vi "9-1.vi"() -> ()   [LabVIEW 2019, in "9.lvlib"]
uses:
  9.lvlib
panel:
  out "number":i32[][](array[numeric])
  out "sum":i32
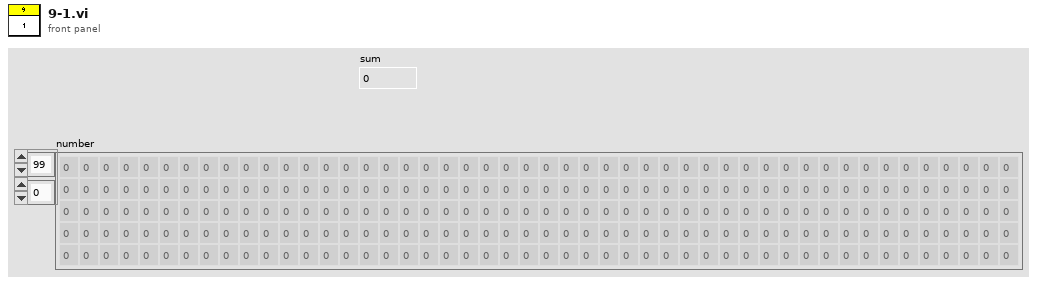
[diagram p1: front panel]
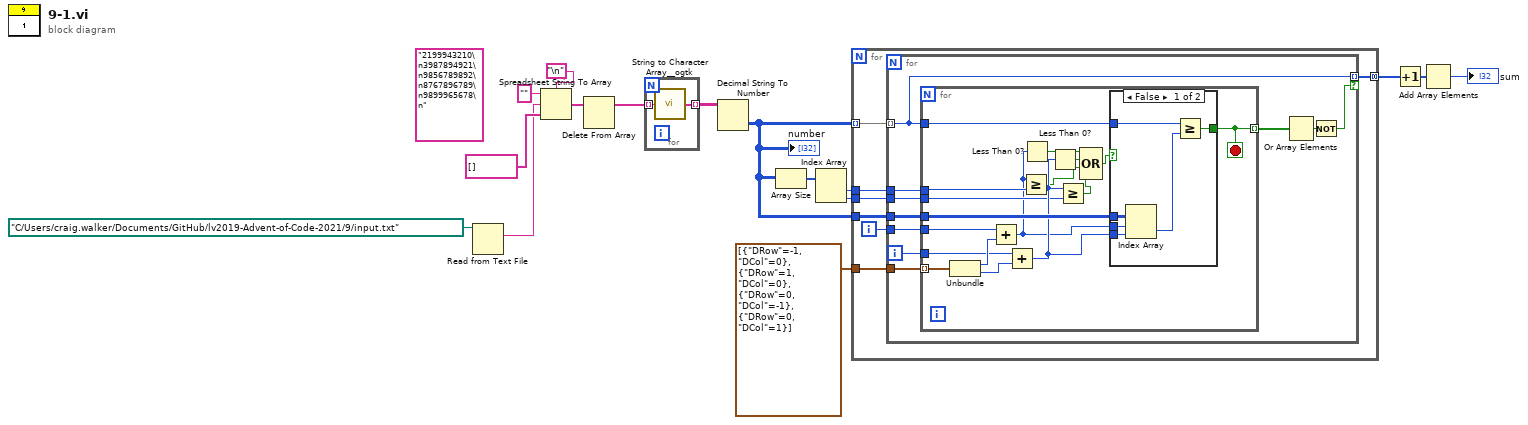
[diagram p0: block diagram]
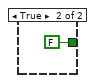
[diagram p2: hidden frame]
diagram:
  (unwired) "2199943210\n3987894921\n9856789892\n8767896789\n9899965678\n"
  n1 = Read from Text File(file (use dialog)=path "C:/Users/craig.walker/Documents/GitHub/lv2019-Advent-of-Code-2021/9/input.txt") -> (text=w1:string)  [unwired: 3 in, 3 out]
  n2 = Spreadsheet String To Array(delimiter (Tab)="\n", format string="", spreadsheet string=w1, array type (2D Dbl)=string[] []) -> (array=w15:string[])
  n3 = Delete From Array(array=w15) -> (array with subset deleted=w2:string[])  [unwired: 2 in, 1 out]
  n4 = for {
    tunnel: w2 -> [w18] mode=indexing
    tunnel: [w17] -> w13 mode=indexing
    n5 = call <userlib>:"String to Character Array__ogtk.vi"("Input String"=w18) -> ("Character Array"=w17:string[])
  }
  n6 = Decimal String To Number(string=w13) -> (number=w3:i32[][])  [unwired: 2 in, 1 out]
  "number" <- w3
  n7 = Array Size(array=w3) -> (size(s)=w7:i32[])
  n8 = Index Array(array=w7) -> (element #1=w9:i32, element #2=w8:i32)  [unwired: 2 in]
  n9 = for {
    tunnel: w3 -> [w24] mode=indexing
    tunnel: w3 -> [w25]
    tunnel: w9 -> [w22]
    tunnel: w8 -> [w21]
    tunnel: cluster{"DRow":i32, "DCol":i32}[] [{"DRow"=-1, "DCol"=0}, {"DRow"=1, "DCol"=0}, {"DRow"=0, "DCol"=-1}, {"DRow"=0, "DCol"=1}] -> [w20]
    tunnel: [w19] -> w12 mode=concatenating
    i -> [w23]
    n10 = for {
      tunnel: w25 -> [w35]
      tunnel: w24 -> [w32] mode=indexing
      tunnel: w23 -> [w28]
      tunnel: w22 -> [w29]
      tunnel: w21 -> [w30]
      tunnel: w20 -> [w34]
      tunnel: [w32] -> w19 mode=indexing if=w26
      i -> [w27]
      n11 = for {
        tunnel: w35 -> [w44]
        tunnel: w28 -> [w50]
        tunnel: w27 -> [w48]
        tunnel: w34 -> [w52] mode=indexing
        tunnel: w32 -> [w42]
        tunnel: [w43] -> w33 mode=indexing
        tunnel: w30 -> [w40]
        tunnel: w29 -> [w39]
        stop <- w43 stop-if-true
        n12 = Unbundle(w52) -> ("DRow"=w51:i32, "DCol"=w49:i32)
        n13 = Add(x=w50, y=w51) -> (x+y=w38:i32)
        n14 = Add(x=w48, y=w49) -> (x+y=w41:i32)
        n15 = Greater Or Equal?(x=w38, y=w39) -> (x >= y?=w37:bool)
        n16 = Less Than 0?(x=w38) -> (x < 0?=w46:bool)
        n17 = Less Than 0?(x=w41) -> (x < 0?=w47:bool)
        n18 = Greater Or Equal?(x=w41, y=w40) -> (x >= y?=w36:bool)
        n19 = Compound Arithmetic op=OR(w46, w47, w37, w36) -> (w45:bool)
        n20 = case shown="False" w45 {
          tunnel: w42 -> [w58 _]
          tunnel: w44 -> [w57 _]
          tunnel: w38 -> [w56 _]
          tunnel: w41 -> [w55 _]
          tunnel: [w53 FALSE] -> w43
          frame False {
            n21 = Index Array(array=w57, index (row)=w56, index (col)=w55) -> (element=w54:i32)
            n22 = Greater Or Equal?(x=w58, y=w54) -> (x >= y?=w53:bool)
          }
          frame True {
          }
        }
      }
      n23 = Or Array Elements(Boolean array=w33) -> (logical OR=w31:bool)
      n24 = Not(x=w31) -> (.not. x?=w26:bool)
    }
  }
  n25 = Increment(x=w12) -> (x+1=w4:i32[])
  n26 = Add Array Elements(numeric array=w4) -> (sum=→"sum":i32)
